vi "Self-Test.vi"(8 "error in":errorcluster, 11 "NI Analog Input in":refnum<class "NI Analog Input.lvclass">) -> (0 "error out":errorcluster, 2 "Result":variant, 3 "NI Analog Input out":refnum<class "NI Analog Input.lvclass">)   [LabVIEW 2020, in "NI Analog Input.lvlib" / "NI Analog Input.lvclass"]
uses:
  NI Analog Input.lvclass
  Utilities/NI SysCfg.lvlib
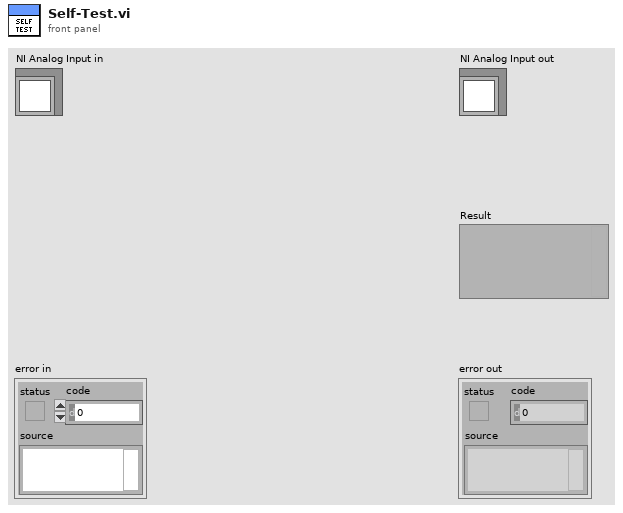
[diagram p1: front panel]
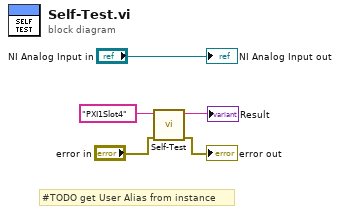
[diagram p0: block diagram]
diagram:
  # "#TODO get User Alias from instance"
  n1 = call "Self-Test.vi"("error in"="error in", "Resource"="PXI1Slot4") -> ("error out"=→"error out":errorcluster, "Result"=→"Result":string)  [unwired: 8 in]
  "NI Analog Input out" <- "NI Analog Input in"
